vi "Target Select with keyboard.vi"(0 "High":bool, 5 "Right":bool, 7 "Left":bool, 9 "Low":bool, 11 "Pyramid":bool) -> (4 "1":bool, 6 "2":bool, 8 "3":bool, 10 "4":bool, 15 "5":bool)   [LabVIEW 2012]
uses:
  Keys Pressed Global.vi
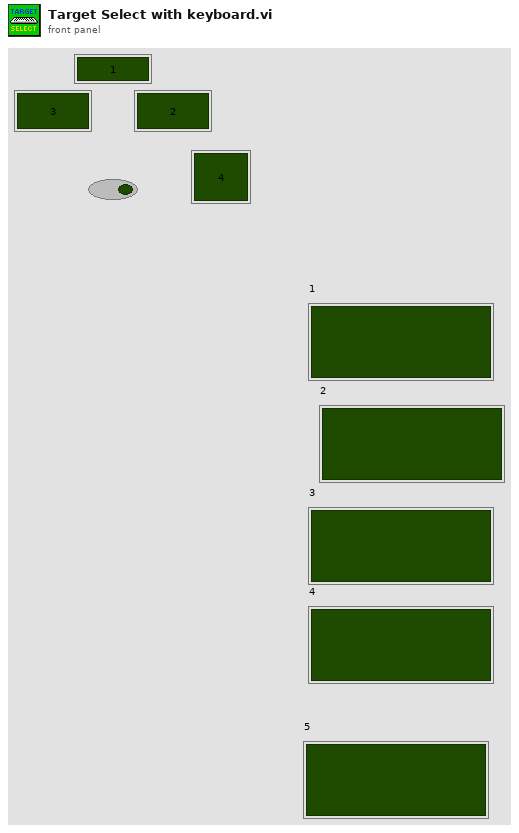
[diagram p1: front panel]
types:
  T1 = enum16{"0", "1", "2", "3", "4", "5", "6", "7", "8", "9", "A", "B", "C", "D", "E", "F", "G", "H", "I", "J", "K", "L", "M", "N", "O", "P", "Q", "R", "S", "T", "U", "V", "W", "X", "Y", "Z", "F1", "F2", "F3", "F4", "F5", "F6", "F7", "F8", "F9", "F10", "F11", "F12", "F13", "F14", "F15", "ADD", "BACK", "BACKSLASH", "CAPITAL", "COMMA", "DECIMAL", "DELETE", "DIVIDE", "DOWN", "END", "EQUALS", "ESCAPE", "GRAVE (`)", "HOME", "INSERT", "LBRACKET", "LCONTROL", "LEFT", "L ALT", "LSHIFT", "LWIN", "MINUS", "MULTIPLY", "NEXT", "NUMLOCK", "NUMPAD_0", "NUMPAD_1", "NUMPAD_2", "NUMPAD_3", "NUMPAD_4", "NUMPAD_5", "NUMPAD_6", "NUMPAD_7", "NUMPAD_8", "NUMPAD_9", "PAUSE", "PERIOD", "PRIOR (PG UP)", "RBRACKET", "RCONTROL", "RETURN", "RIGHT", "R ALT", "RSHIFT", "RWIN", "SCROLL", "SEMICOLON", "SLASH", "SPACE", "SUBTRACT", "TAB", "UP", "ENTER (num pad)", "' (quote)"}
  T2 = enum16{"0", "1", "2", "3", "4", "5", "6", "7", "8", "9", "A", "B", "C", "D", "E", "F", "G", "H", "I", "J", "K", "L", "M", "N", "O", "P", "Q", "R", "S", "T", "U", "V", "W", "X", "Y", "Z", "F1", "F2", "F3", "F4", "F5", "F6", "F7", "F8", "F9", "F10", "F11", "F12", "F13", "F14", "F15", "ADD", "BACK", "BACKSLASH", "CAPITAL", "COMMA", "DECIMAL", "DELETE", "DIVIDE", "DOWN", "END", "EQUALS", "ESCAPE", "GRAVE (`)", "HOME", "INSERT", "LBRACKET", "LCONTROL", "LEFT", "L ALT", "LSHIFT", "LWIN", "MINUS", "MULTIPLY", "NEXT", "NUMLOCK", "NUMPAD_0", "NUMPAD_1", "NUMPAD_2", "NUMPAD_3", "NUMPAD_4", "NUMPAD_5", "NUMPAD_6", "NUMPAD_7", "NUMPAD_8", "NUMPAD_9", "PAUSE", "PERIOD", "PRIOR (PG UP)", "RBRACKET", "RCONTROL", "RETURN", "RIGHT", "R ALT", "RSHIFT", "RWIN", "SCROLL", "SEMICOLON", "SLASH", "SPACE", "SUBTRACT", "TAB", "UP", "ENTER (num pad)", "' (quote)"}[]
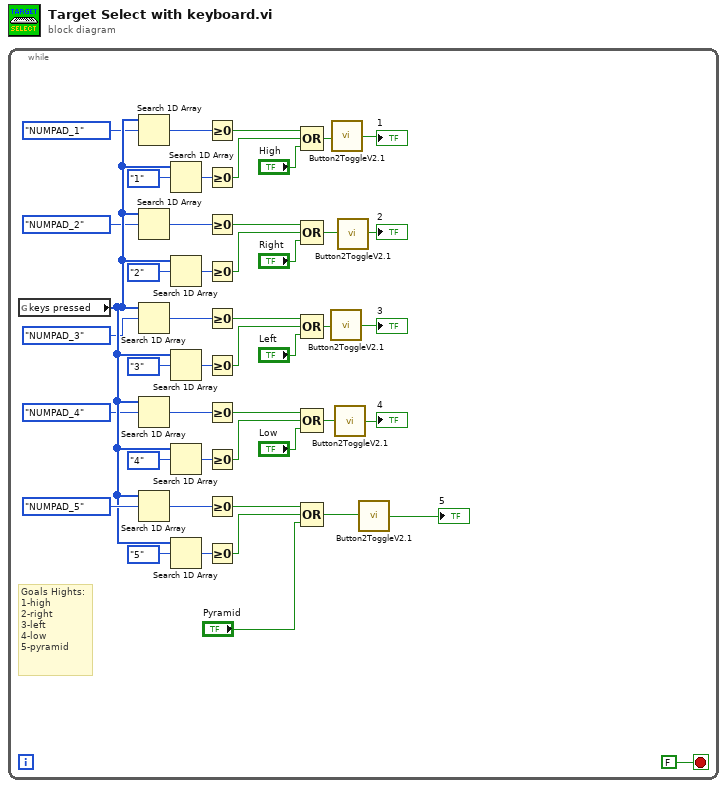
[diagram p0: block diagram]
diagram:
  n1 = while {
    stop <- FALSE stop-if-true
    # "Goals Hights:\n1-high\n2-right\n3-left\n4-low\n5-pyramid"
    n2 = global read "Keys Pressed Global.vi" "keys pressed"() -> (w40:T2)
    n3 = Search 1D Array(1D array=w40, element=T1."NUMPAD_1" ("keys pressed[0]")) -> (index of element=w23:i32)  [unwired: 1 in]
    n4 = Search 1D Array(1D array=w40, element=T1."NUMPAD_2" ("keys pressed[0]")) -> (index of element=w30:i32)  [unwired: 1 in]
    n5 = Search 1D Array(1D array=w40, element=T1."NUMPAD_3" ("keys pressed[0]")) -> (index of element=w31:i32)  [unwired: 1 in]
    n6 = Search 1D Array(1D array=w40, element=T1."NUMPAD_4" ("keys pressed[0]")) -> (index of element=w38:i32)  [unwired: 1 in]
    n7 = Search 1D Array(1D array=w40, element=T1."NUMPAD_5" ("keys pressed[0]")) -> (index of element=w41:i32)  [unwired: 1 in]
    n8 = Search 1D Array(1D array=w40, element=T1."1" ("keys pressed[0]")) -> (index of element=w26:i32)  [unwired: 1 in]
    n9 = Search 1D Array(1D array=w40, element=T1."2" ("keys pressed[0]")) -> (index of element=w27:i32)  [unwired: 1 in]
    n10 = Search 1D Array(1D array=w40, element=T1."3" ("keys pressed[0]")) -> (index of element=w34:i32)  [unwired: 1 in]
    n11 = Search 1D Array(1D array=w40, element=T1."4" ("keys pressed[0]")) -> (index of element=w35:i32)  [unwired: 1 in]
    n12 = Search 1D Array(1D array=w40, element=T1."5" ("keys pressed[0]")) -> (index of element=w44:i32)  [unwired: 1 in]
    n13 = Greater Or Equal To 0?(x=w23) -> (x >= 0?=w22:bool)
    n14 = Greater Or Equal To 0?(x=w26) -> (x >= 0?=w21:bool)
    n15 = Greater Or Equal To 0?(x=w30) -> (x >= 0?=w19:bool)
    n16 = Greater Or Equal To 0?(x=w27) -> (x >= 0?=w18:bool)
    n17 = Greater Or Equal To 0?(x=w31) -> (x >= 0?=w16:bool)
    n18 = Greater Or Equal To 0?(x=w34) -> (x >= 0?=w15:bool)
    n19 = Greater Or Equal To 0?(x=w38) -> (x >= 0?=w14:bool)
    n20 = Greater Or Equal To 0?(x=w35) -> (x >= 0?=w13:bool)
    n21 = Greater Or Equal To 0?(x=w41) -> (x >= 0?=w45:bool)
    n22 = Greater Or Equal To 0?(x=w44) -> (x >= 0?=w46:bool)
    n23 = Compound Arithmetic op=OR(w22, w21, "High") -> (w7:bool)
    n24 = Compound Arithmetic op=OR(w19, w18, "Right") -> (w8:bool)
    n25 = Compound Arithmetic op=OR(w16, w15, "Left") -> (w9:bool)
    n26 = Compound Arithmetic op=OR(w14, w13, "Low") -> (w10:bool)
    n27 = Compound Arithmetic op=OR(w45, w46, "Pyramid") -> (w1:bool)
    n28 = call "Button2ToggleV2.1.vi"("a"=w9) -> ("Result(clone)"=→"3":bool)
    n29 = call "Button2ToggleV2.1.vi"("a"=w7) -> ("Result(clone)"=→"1":bool)
    n30 = call "Button2ToggleV2.1.vi"("a"=w10) -> ("Result(clone)"=→"4":bool)
    n31 = call "Button2ToggleV2.1.vi"("a"=w8) -> ("Result(clone)"=→"2":bool)
    n32 = call "Button2ToggleV2.1.vi"("a"=w1) -> ("Result(clone)"=→"5":bool)
  }
